vi "Go to field (PID).vi"(8 "error in (no error)":errorcluster, 10 "Desired Field":dbl[unit], 11 "Varian Magnet.lvclass In":refnum<class "Varian Magnet.lvclass">) -> (0 "error out":errorcluster, 1 "Control Voltage":dbl, 2 "Current Field":dbl[unit], 3 "Varian Magnet out":refnum<class "Varian Magnet.lvclass">)   [LabVIEW 2009, in "Varian Magnet.lvclass"]
doc: "Uses a PID controller to maintain field at desired value. Uses last 5 field points from member data to record previous points."
uses:
  Varian Magnet.lvclass
  Varian Magnet.lvclass/Varian Magnet.ctl
  Varian/Varian.lvlib
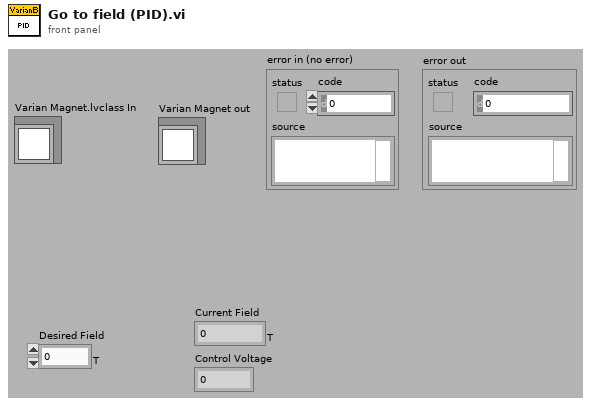
[diagram p1: front panel]
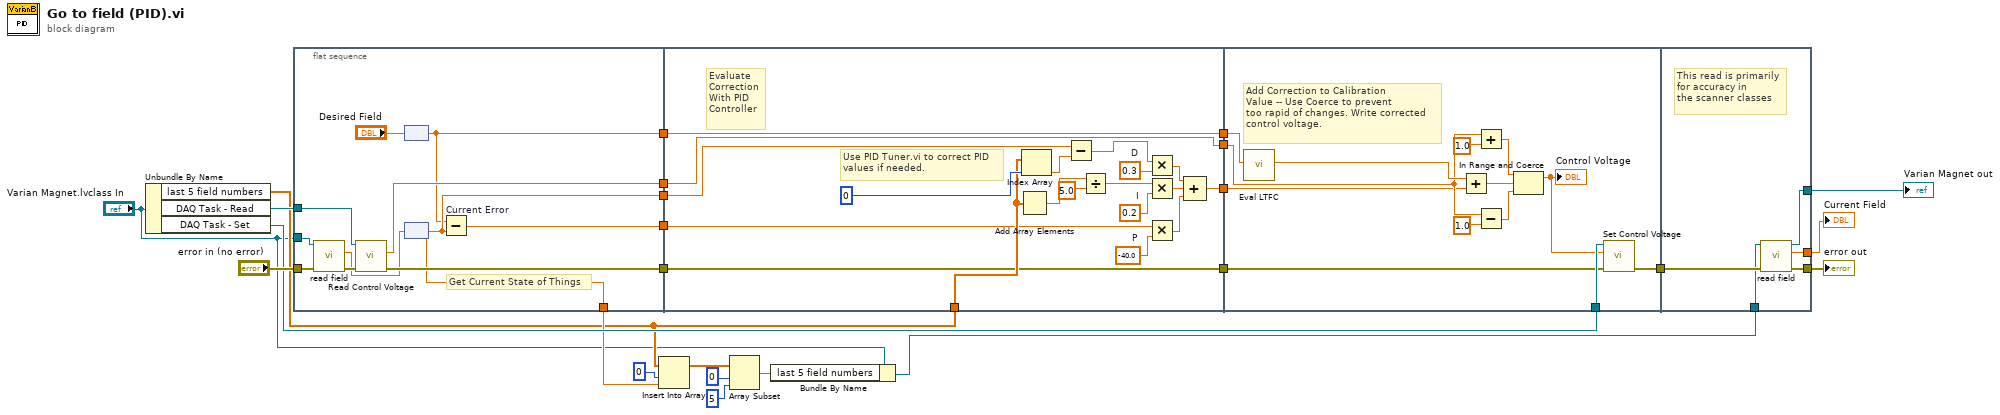
[diagram p0: block diagram]
diagram:
  n1 = Unbundle By Name("Varian Magnet.lvclass In") -> ("last 5 field numbers"=w11:dbl[], "DAQ Task - Read"=w20:refnum<k21>, "DAQ Task - Set"=w16:refnum<k21>)
  n2 = flat-sequence {
    tunnel: "Varian Magnet.lvclass In" -> [w36]
    tunnel: "error in (no error)" -> [w35]
    tunnel: [w34] -> w24
    tunnel: [w29] -> w23
    tunnel: [w28] -> w21
    tunnel: w20 -> [w32]
    tunnel: [w31] -> w18
    tunnel: [w30] -> w14
    tunnel: [w29] -> w13
    tunnel: w11 -> [w52]
    tunnel: w24 -> [w49]
    tunnel: w23 -> [w50]
    tunnel: [w40] -> w22
    tunnel: w21 -> [w40]
    tunnel: [w39] -> w19
    tunnel: w18 -> [w39]
    tunnel: [w38] -> w17
    tunnel: [w37] -> w15
    tunnel: w14 -> [w37]
    tunnel: w22 -> [w68]
    tunnel: w19 -> [w65]
    tunnel: w17 -> [w60]
    tunnel: w16 -> [w59]
    tunnel: w15 -> [w58]
    tunnel: [w57] -> w5
    tunnel: w5 -> [w73]
    tunnel: [w72] -> w4
    tunnel: w3 -> [w71]
    tunnel: [w70] -> w2
    tunnel: [w69] -> w1
    frame #0 {
      # "Get Current State of Things"
      n3 = call "read field.vi"("error in (no error)"=w35, "Varian Magnet.lvclass In"=w36) -> ("error out"=w33:errorcluster, "Field"=w26:dbl[unit])  [unwired: 7 in, 1 out]
      n4 = call "Read Control Voltage.vi"("error in"=w33, "task in"=w32) -> ("error out"=w30:errorcluster, "Current Control Voltage"=w31:dbl)  [unwired: 7 in, 1 out]
      n5 = node("Desired Field") -> (w28:dbl)
      n6 = node(w26) -> (w29:dbl)
      n7 = Subtract "Current Error"(x=w28, y=w29) -> (x-y=w34:dbl)
    }
    frame #1 {
      w48 = -40.0  # P
      w44 = 0.3  # D
      w46 = 0.2  # I
      # "Use PID Tuner.vi to correct PID\nvalues if needed."
      # "Evaluate\nCorrection\nWith PID\nController"
      n8 = Add Array Elements(numeric array=w52) -> (sum=w55:dbl)
      n9 = Index Array(array=w52, index=0) -> (element=w54:dbl)
      n10 = Subtract(x=w50, y=w54) -> (x-y=w45:dbl)
      n11 = Divide(x=w55, y=5.0) -> (x/y=w47:dbl)
      n12 = Multiply(x=w45, y=w44) -> (x*y=w43:dbl)
      n13 = Multiply(x=w47, y=w46) -> (x*y=w42:dbl)
      n14 = Multiply(x=w49, y=w48) -> (x*y=w41:dbl)
      n15 = Compound Arithmetic op=ADD(w43, w42, w41) -> (w38:dbl)
    }
    frame #2 {
      # "Add Correction to Calibration\nValue -- Use Coerce to prevent\ntoo rapid of changes. Write corrected\ncontrol voltage."
      n16 = call "Eval LTFC.vi"("Desired Field (T)"=w68) -> ("Desired Control Voltage"=w67:dbl)  [unwired: 9 in, 1 out]
      n17 = Add(x=w67, y=w60) -> (x+y=w66:dbl)
      n18 = Add(x=w65, y=1.0) -> (x+y=w61:dbl)
      n19 = Subtract(x=w65, y=1.0) -> (x-y=w62:dbl)
      n20 = In Range and Coerce(upper limit=w61, x=w66, lower limit=w62) -> (coerced(x)=w56:dbl)  [unwired: 1 out]
      "Control Voltage" <- w56
      n21 = call "Set Control Voltage.vi"("error in"=w58, "Control Voltage"=w56, "task in"=w59) -> ("error out"=w57:errorcluster)  [unwired: 8 out]
    }
    frame #3 {
      # "This read is primarily\nfor accuracy in\nthe scanner classes"
      n22 = call "read field.vi"("error in (no error)"=w73, "Varian Magnet.lvclass In"=w71) -> ("error out"=w72:errorcluster, "Field"=w69:dbl[unit], "Varian Magnet.lvclass Out"=w70:refnum<class "Varian Magnet.lvclass">)  [unwired: 7 in]
    }
  }
  n23 = Insert Into Array(array=w11, index=0, new element=w13) -> (w10:dbl[])
  n24 = Array Subset(array=w10, index=0, length=5) -> (w6:dbl[])
  n25 = Bundle By Name(cluster="Varian Magnet.lvclass In", "last 5 field numbers"=w6) -> (w3:refnum<class "Varian Magnet.lvclass">)
  "Varian Magnet out" <- w2
  "error out" <- w4
  "Current Field" <- w1
